vi "Add Library to Project.vi"(8 "error in":errorcluster, 10 "plugin library path":path, 11 "project refnum":refnum<vi>) -> (0 "error out":errorcluster)   [LabVIEW 2021, in "InstrumentStudio Plug-In Editor.lvlib"]
uses:
  InstrumentStudio Plug-In Editor.lvlib
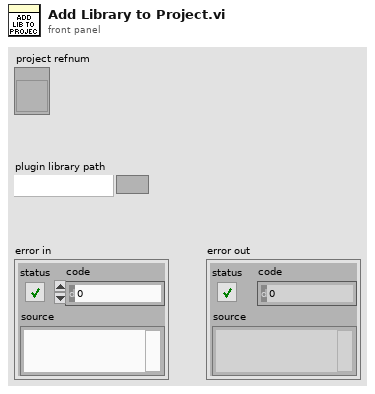
[diagram p1: front panel]
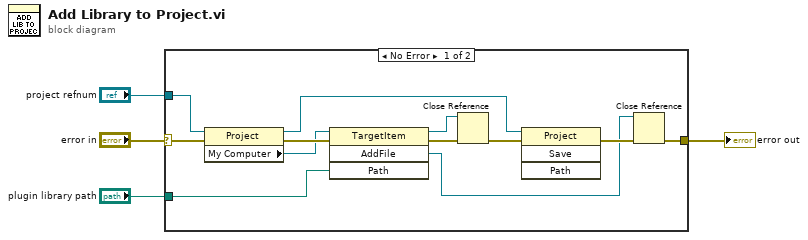
[diagram p0: block diagram]
diagram:
  n1 = case shown="No Error" "error in" {
    selector: "error in" -> [w11 w17]
    tunnel: "plugin library path" -> [w6 _]
    tunnel: "project refnum" -> [w10 _]
    tunnel: [w8 w17] -> w1
    frame No Error {
      n2 = property class="Project"(reference=w10, error in=w11) -> (reference out=w16:refnum<vi>, error out=w13:errorcluster, "My Computer"=w12:refnum<vi>)
      n3 = invoke class="TargetItem" method="AddFile"(reference=w12, error in=w13, "Path"=w6) -> (reference out=w5:refnum<vi>, error out=w14:errorcluster, "AddFile"=w7:refnum<vi>)  [unwired: 1 in, 1 out]
      n4 = Close Reference(reference=w5, error in (no error)=w14) -> (error out=w15:errorcluster)
      n5 = invoke class="Project" method="Save"(reference=w16, error in=w15) -> (error out=w9:errorcluster)  [unwired: 2 in, 3 out]
      n6 = Close Reference(reference=w7, error in (no error)=w9) -> (error out=w8:errorcluster)
    }
    frame Error {
    }
  }
  "error out" <- w1
